vi "Sort Archive Records.vi"(0 "Text":cluster{"Records":string[]}[](array[cluster]), 1 "Number of\nLBCBs In":T2, 2 "2 LBCB Archiving Mode":bool) -> (4 "Sorted Records":string[](array[string]))   [LabVIEW 2009]
uses:
  Data Access Objects/Application/Number Of LBCBs.ctl
  Archive File Type.ctl
panel:
  in  "Archive File Type":T1
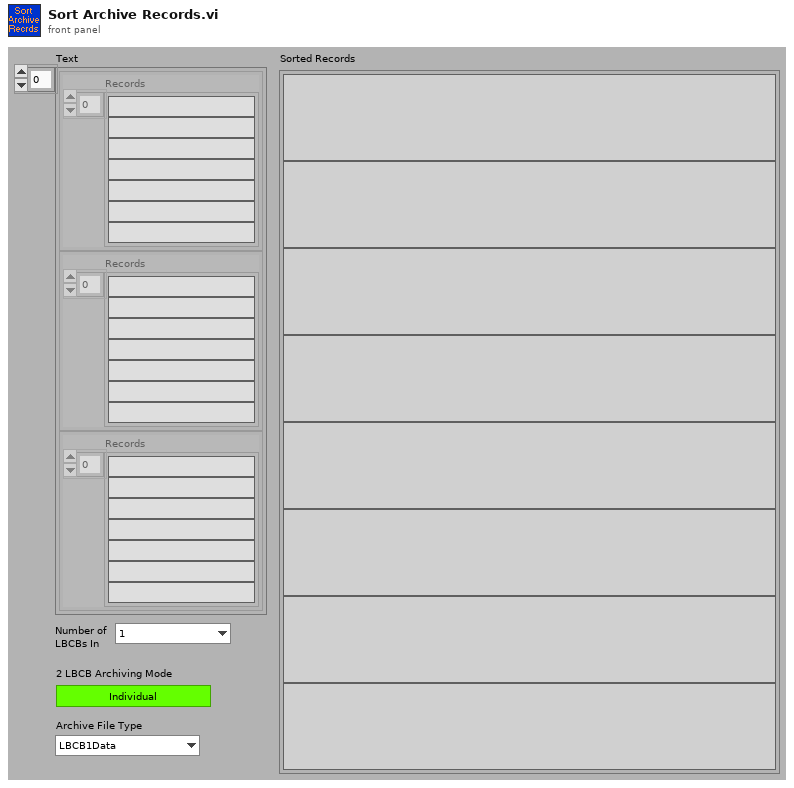
[diagram p1: front panel]
types:
  T1 = typedef "Archive File Type.ctl" = enum16{"LBCB1Data", "LBCB2Data", "ExternalSensors", "CombinedData", "LBCB1Commands", "LBCB2Commands", "CombinedCommands", "LBCB1Stiffness", "LBCB2Stiffness", "CombinedStiffness"}
  T2 = typedef "Number Of LBCBs.ctl" = enum16{"1", "2"}
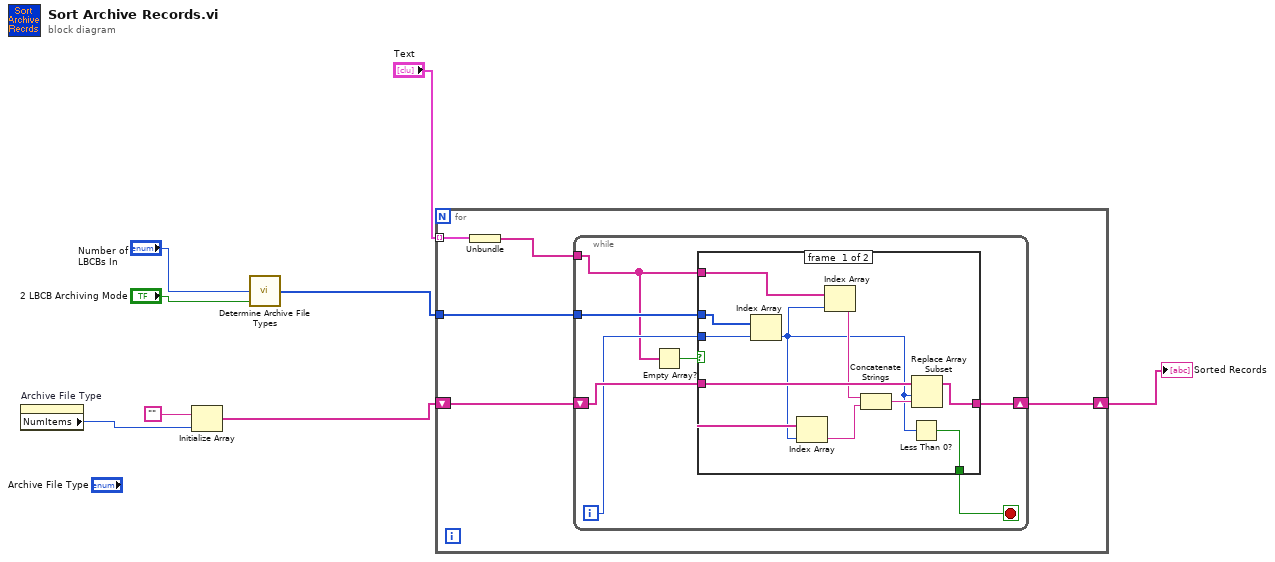
[diagram p0: block diagram]
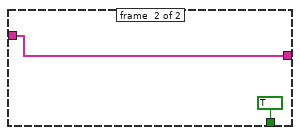
[diagram p2: hidden frame]
diagram:
  n1 = property on="Archive File Type" class="Enum (strict)"() -> ("NumItems"=w3:u32)  [unwired: 2 in, 2 out]
  n2 = Initialize Array("", w3) -> (w2:string[])
  n3 = call "Determine Archive File Types.vi"("2 LBCB Archiving Mode"="2 LBCB Archiving Mode", "Number of\nLBCBs In"="Number of\nLBCBs In") -> ("File Type Indexes"=w5:i32[])  [unwired: 1 in]
  n4 = for {
    tunnel: "Text" -> [w13] mode=indexing
    tunnel: w5 -> [w11]
    shift-right: [w9] -> w1
    shift-left: w2 -> [w10]
    n5 = Unbundle(w13) -> ("Records"=w12:string[])
    n6 = while {
      tunnel: w12 -> [w14]
      tunnel: w11 -> [w20]
      shift-right: [w17] -> w9
      shift-left: w10 -> [w18]
      i -> [w16]
      stop <- w19 stop-if-true
      n7 = Empty Array?(array=w14) -> (empty?=w15:bool)
      n8 = case shown="False" w15 {
        tunnel: w20 -> [w30 _]
        tunnel: [w29 TRUE] -> w19
        tunnel: w14 -> [w28 _]
        tunnel: w18 -> [w26 w32]
        tunnel: [w24 w32] -> w17
        tunnel: w16 -> [w22 _]
        frame #0 {
          n9 = Index Array(array=w30, index=w22) -> (element=w21:i32)
          n10 = Index Array(array=w26, index=w21) -> (element=w27:string)
          n11 = Index Array(array=w28, index=w21) -> (element=w23:string)
          n12 = Concatenate Strings(w23, w27) -> (w25:string)
          n13 = Less Than 0?(x=w21) -> (x < 0?=w29:bool)
          n14 = Replace Array Subset(array=w26, new element=w25, index=w21) -> (w24:string[])
        }
        frame #1 {
        }
      }
    }
  }
  "Sorted Records" <- w1
